vi "Loop_SM.vi"() -> ()   [LabVIEW 2017]
uses:
  ENUM_SM_State.ctl
  ENUM_SM_Action.ctl
  TypeDef/CLUSTER_CMD_WC_Drive.ctl
  TypeDef/ENUM_WC_Drive_DriveMode.ctl
  TypeDef/CLUSTER_Drive_ACT Loop_VBus Data.ctl
  TypeDef/CLUSTER_X and Y.ctl
  TypeDef/CLUSTER_Drive_ACT Loop_Profile Data.ctl
  TypeDef/CLUSTER_Left and Right.ctl
  TypeDef/ENUM_Drive_ACT Loop_Mode.ctl
  TypeDef/CLUSTER_Drive_HW_SRX_Status.ctl
  TypeDef/CLUSTER_4296_SRX_Status.ctl
  TypeDef/CLUSTER_SRX_Status Data.ctl
  TypeDef/CLUSTER_SRX_Encoder Data.ctl
  TypeDef/CLUSTER_SRX_PWM Data.ctl
  TypeDef/CLUSTER_SRX_Analog Data.ctl
  TypeDef/CLUSTER_SRX_Limit Switch Data.ctl
  TypeDef/CLUSTER_SRX_Profile Data.ctl
  <vilib>/Rock Robotics/WPI/ThirdParty/Sensors/navX/_TypeDefs/FRIC_navX_DeviceNumbersTypeDef.ctl
  _SHARE ALL/Global Share All/Global_STOP.vi
  Globals/Global_CMD_Drive.vi
  Global_ACT Write_Data Out.vi
  <vilib>/addons/control/pid/pid.llb/PID (DBL).vi
  Global_SM Write_Data Out.vi
  <vilib>/addons/control/pid/NI_PID_pid.lvlib
panel:
  in  "PID gains Cube Follow":T1={"proportional gain (Kc)"=0.01, "integral time (Ti, min)"=0.0, "derivative time (Td, min)"=0.0} {"derivative time (Td, min)" format="%.3f"; "integral time (Ti, min)" format="%.3f"; "proportional gain (Kc)" format="%.8f"}
  in  "Pixel allowence":dbl=10.0 format="%#_13g"
  in  "Degree allowence":dbl=2.0 format="%#_13g"
  in  "PID gains Lock Angle":T1={"proportional gain (Kc)"=0.01, "integral time (Ti, min)"=0.0, "derivative time (Td, min)"=0.0} {"derivative time (Td, min)" format="%.3f"; "integral time (Ti, min)" format="%.3f"; "proportional gain (Kc)" format="%.8f"}
  in  "MAX sensativity":dbl=1.0
  in  "Max RPM":dbl=10000.0
  in  "MIN sensativity":dbl=0.2
  out "Cycle Time (S)":dbl format="%.3g"
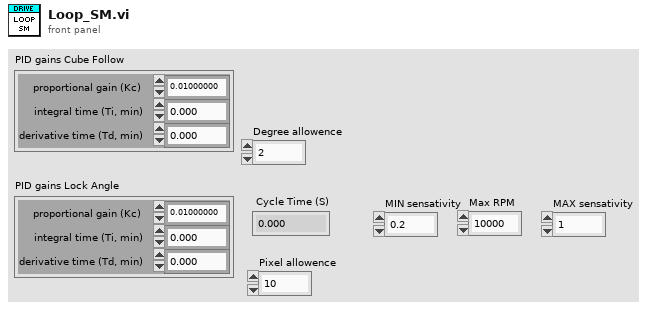
[diagram p1: front panel]
types:
  T1 = cluster{"proportional gain (Kc)":dbl, "integral time (Ti, min)":dbl, "derivative time (Td, min)":dbl}
  T2 = cluster{"Rollover":dbl, "Yaw":dbl, "Cont Yaw":dbl}
  T3 = typedef "CLUSTER_Drive_HW_SRX_Status.ctl" = cluster{"Rear Left":T4, "Rear Right":T4, "Front Left":T4, "Front Right":T4}
  T4 = typedef "CLUSTER_4296_SRX_Status.ctl" = cluster{"Status":T5, "Encoder":T6, "PWM ":T7, "Analog":T8, "Limit Switches":T9, "Profile":T10}
  T5 = typedef "CLUSTER_SRX_Status Data.ctl" = cluster{"Module Enabled":bool, "Current Profile Slot Select":dbl, "Brake is Enabled":bool, "Applied Throttle":dbl, "Current":dbl, "Battery Voltage":dbl, "Sticky Fault - Under Voltage":bool, "Temperature (C)":dbl, "Sticky Fault - Over Temp":bool, "CAN Error":errorcluster, "Control 5 Is Supported":bool}
  T6 = typedef "CLUSTER_SRX_Encoder Data.ctl" = cluster{"Closed Loop Error":dbl, "Sensor Position":dbl, "Sensor Velocity":dbl, "Encoder Position":dbl, "Encoder Velocity":dbl, "Encoder Index Count":dbl, "Encoder A Pin State":bool, "Encoder B Pin State":bool, "Encoder Index Pin State":bool, "Pos Div 8":bool, "Vel Div 4":bool}
  T7 = typedef "CLUSTER_SRX_PWM Data.ctl" = cluster{"Closed Loop Error":dbl, "Pulse Width Position":i32, "Pulse Width Velocity":i32, "Pulse Width Rise To Rise (us)":i32, "Pulse Width Rise To Fall (us)":i32}
  T8 = typedef "CLUSTER_SRX_Analog Data.ctl" = cluster{"Closed Loop Error":dbl, "Analog In":dbl, "Analog In Velocity":dbl}
  T9 = typedef "CLUSTER_SRX_Limit Switch Data.ctl" = cluster{"Forward Limit Switch Closed":bool, "Reverse Limit Switch Closed":bool, "Sticky Fault - Forward Limit":bool, "Sticky Fault - Reverse Limit":bool, "Sticky Fault - Forward Soft Limit":bool, "Sticky Fault - Reverse Soft Limit":bool}
  T10 = typedef "CLUSTER_SRX_Profile Data.ctl" = cluster{"Mot Prof Active Is Under Run":bool, "Mot Prof Active Has Under Run":bool, "Mot Prof Active Is Last":bool, "Mot Prof Active Velocity Only":bool, "Mot Prof Active Is Valid":bool, "Mot Prof Buffer Is Full":bool, "Mot Prof Active Profile Slot Select":i32, "Mot Prof NextID":i32, "Mot Prof Count":i32, "Mot Prof Active Velocity":dbl, "Mot Prof Active Position":dbl, "Mot Prof Output Enable":i32}
  T11 = typedef "ENUM_Drive_ACT Loop_Mode.ctl" = enum16{"Stop", "Position", "VBus", "Profile"}
  T12 = typedef "CLUSTER_Left and Right.ctl" = cluster{"Left":dbl, "Right":dbl}
  T13 = typedef "CLUSTER_CMD_WC_Drive.ctl" = cluster{"Drive_Mode":T14, "VBus":T15, "Profile":T17, "Zero Drive Encoders":bool, "Set Target Position(IN)":dbl, "Target Angle(Degree)":dbl, "Lock Angle":bool, "Zero YAW":bool, "Follow Cubes":bool}
  T14 = typedef "ENUM_WC_Drive_DriveMode.ctl" = enum16{"Motion Profile", "CrossLineAuto", "VBus", "Stop"}
  T15 = typedef "CLUSTER_Drive_ACT Loop_VBus Data.ctl" = cluster{"Drive":T16, "Turbo":bool}
  T16 = typedef "CLUSTER_X and Y.ctl" = cluster{"Steer":dbl, "Throtle":dbl}
  T17 = typedef "CLUSTER_Drive_ACT Loop_Profile Data.ctl" = cluster{"Start":bool}
  T18 = typedef "ENUM_SM_Action.ctl" = enum16{"No Action", "Reset Time", "Reset All", "Drive", "Zero YAW", "Shift", "Calculate Sensitivity"}
  T19 = typedef "ENUM_SM_State.ctl" = enum16{"Startup", "VBus", "VBus Lock Angle", "Idle", "Follow Cube", "Shutdown"}
  T20 = cluster{"Action":T18, "State":T19, "Previous State":T19, "Current Time":timestamp, "Previous Time":timestamp, "Start Time":timestamp, "Target Time (ms)":u32, "Cycle Time(S)":dbl, "CMD_Drive":T13, "VBus Output":T12, "Mode Output":T11, "MQuickStopAccumulator":dbl, "SRX_Status":T3, "Sensitivity":dbl, "NavX Yaw":cluster{"Rollover":dbl, "Yaw":dbl, "Cont Yaw":dbl}, "LockAngle":bool, "Zero YAW":bool, "Target Cube Position (Pixels)":dbl, "Follow Cube":bool}
  T21 = typedef "FRIC_navX_DeviceNumbersTypeDef.ctl" = enum16{"Dev0", "Dev1", "Dev2", "Dev3"}
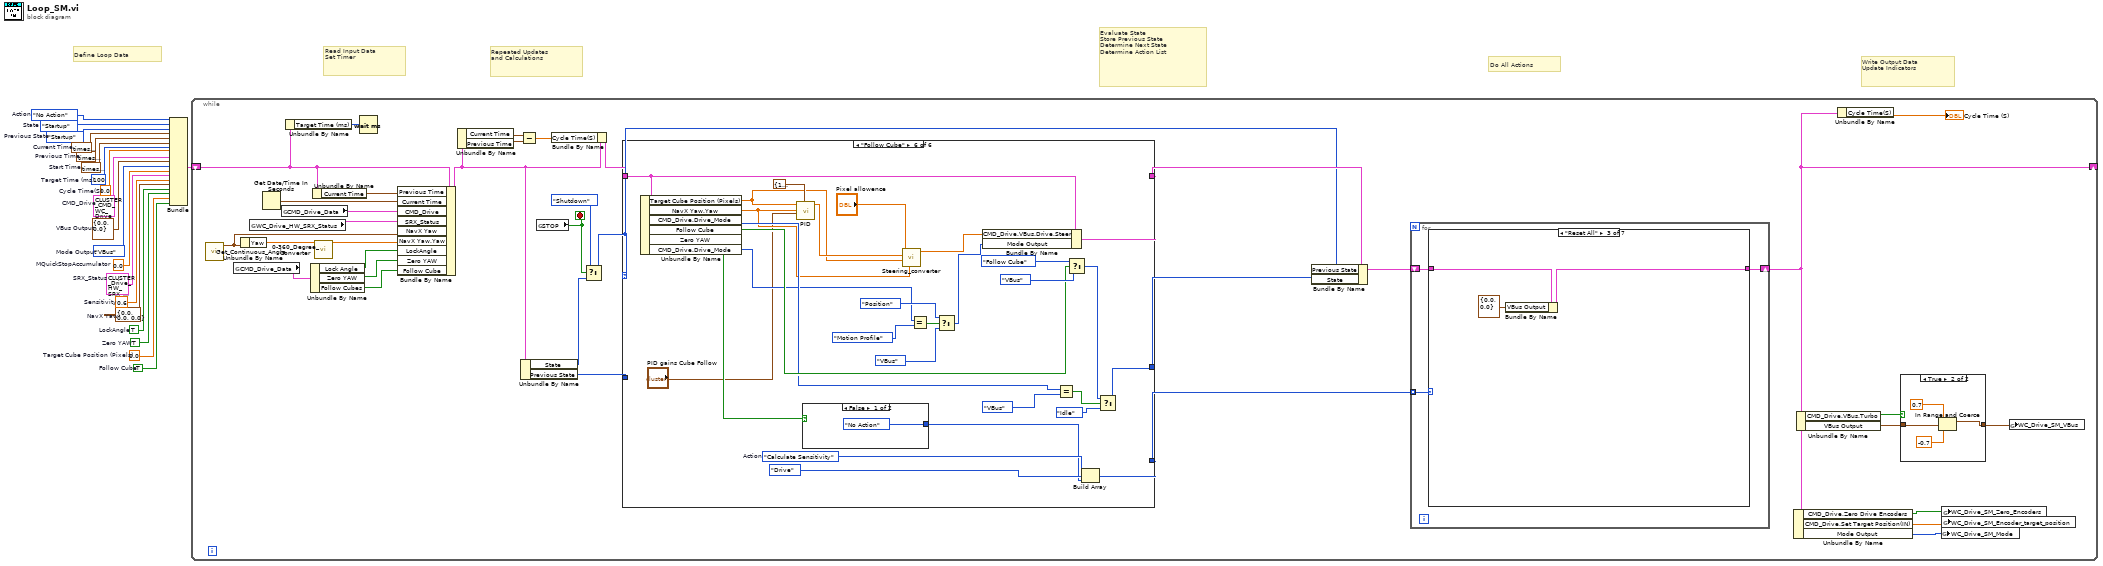
[diagram p0: block diagram]
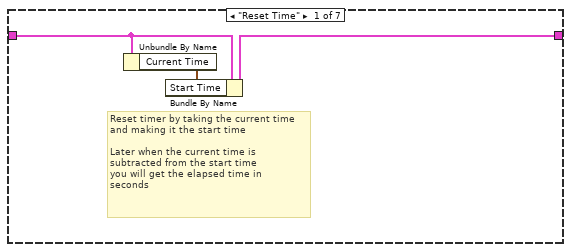
[diagram p3: hidden frame]
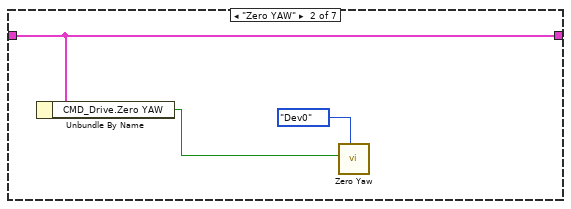
[diagram p4: hidden frame]
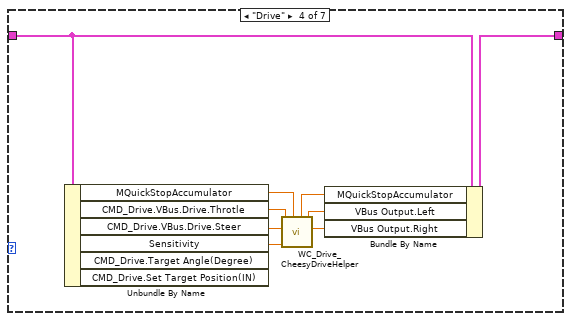
[diagram p5: hidden frame]
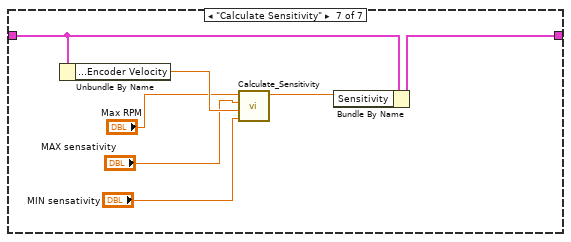
[diagram p8: hidden frame]
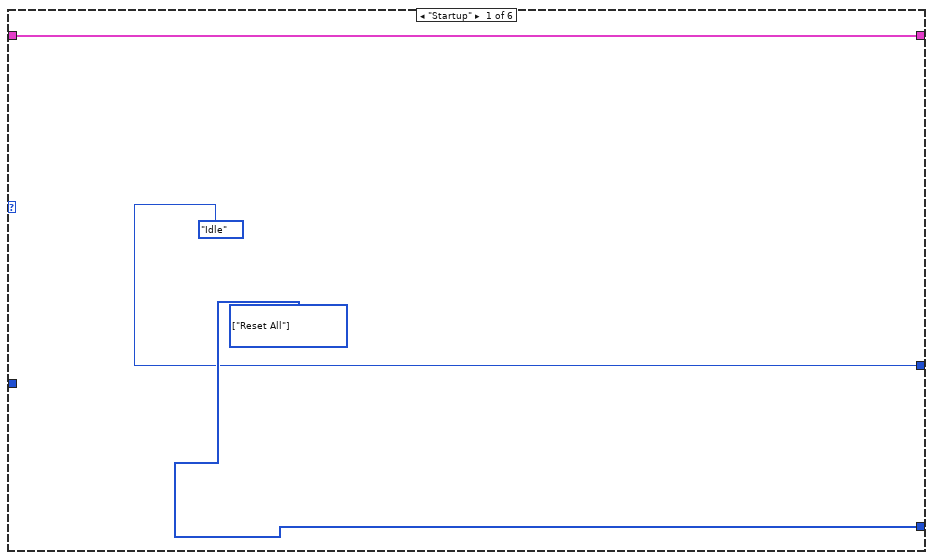
[diagram p9: hidden frame]
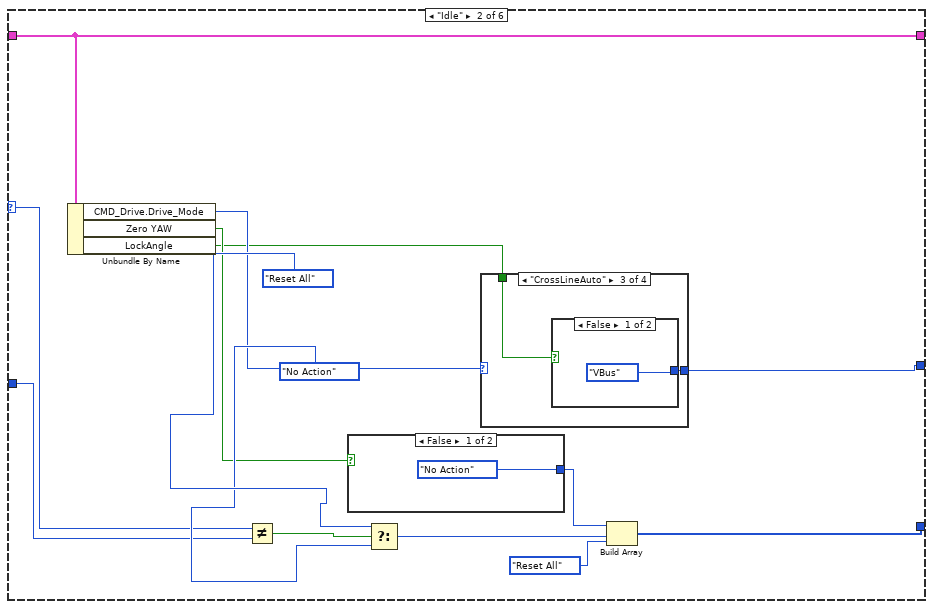
[diagram p10: hidden frame]
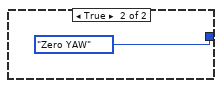
[diagram p11: hidden frame]
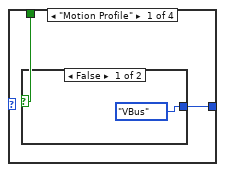
[diagram p12: hidden frame]
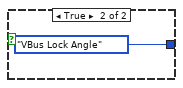
[diagram p13: hidden frame]
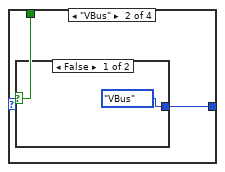
[diagram p14: hidden frame]
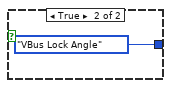
[diagram p15: hidden frame]
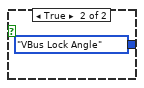
[diagram p16: hidden frame]
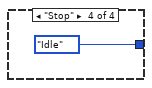
[diagram p17: hidden frame]
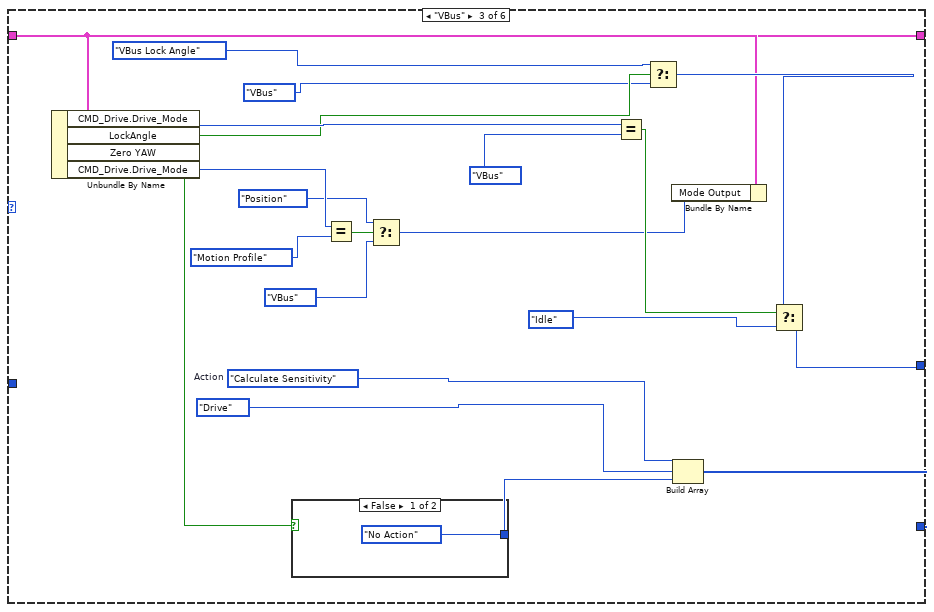
[diagram p18: hidden frame]
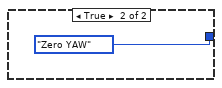
[diagram p19: hidden frame]
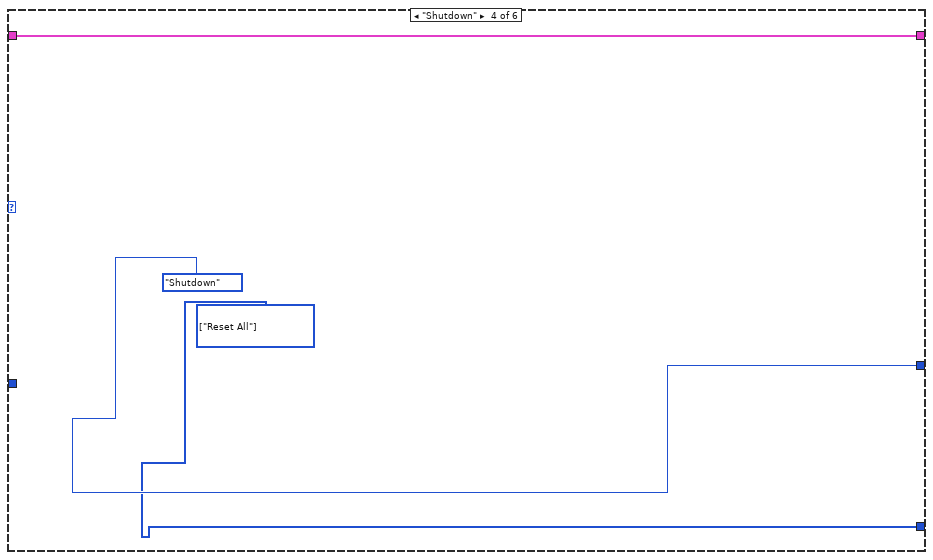
[diagram p20: hidden frame]
diagram:
  w1 = TRUE  # Follow Cube
  w2 = 0.0  # Target Cube Position (Pixels)
  w3 = TRUE  # Zero YAW
  w4 = TRUE  # LockAngle
  w5 = T2 {"Rollover"=0.0, "Yaw"=0.0, "Cont Yaw"=0.0}  # NavX Yaw
  w6 = 0.6  # Sensitivity
  w7 = T3 {"Rear Left"={"Status"={"Module Enabled"=FALSE, "Current Profile Slot Select"=0.0, "Brake is Enabled"=TRUE, "Applied Throttle"=0.0, "Current"=0.0, "Battery Voltage"=12.450000000000001, "Sticky Fault - Under Voltage"=TRUE, "Temperature (C)"=30.645161290322577, "Sticky Fault - Over Temp"=FALSE, "CAN Error"={"status"=FALSE, "code"=0, "source"=""}, "Control 5 Is Supported"=TRUE}, "Encoder"={"Closed Loop Error"=0.0, "Sensor Position"=-847.859619140625, "Sensor Velocity"=0.0, "Encoder Position"=-3472833.0, "Encoder Velocity"=0.0, "Encoder Index Count"=-9452.0, "Encoder A Pin State"=FALSE, "Encoder B Pin State"=FALSE, "Encoder Index Pin State"=FALSE, "Pos Div 8"=FALSE, "Vel Div 4"=FALSE}, "PWM "={"Closed Loop Error"=0.0, "Pulse Width Position"=-3472224, "Pulse Width Velocity"=0, "Pulse Width Rise To Rise (us)"=4187, "Pulse Width Rise To Fall (us)"=1210}, "Analog"={"Closed Loop Error"=0.0, "Analog In"=105.0, "Analog In Velocity"=0.0}, "Limit Switches"={"Forward Limit Switch Closed"=FALSE, "Reverse Limit Switch Closed"=FALSE, "Sticky Fault - Forward Limit"=FALSE, "Sticky Fault - Reverse Limit"=TRUE, "Sticky Fault - Forward Soft Limit"=FALSE, "Sticky Fault - Reverse Soft Limit"=FALSE}, "Profile"={"Mot Prof Active Is Under Run"=FALSE, "Mot Prof Active Has Under Run"=FALSE, "Mot Prof Active Is Last"=FALSE, "Mot Prof Active Velocity Only"=FALSE, "Mot Prof Active Is Valid"=FALSE, "Mot Prof Buffer Is Full"=FALSE, "Mot Prof Active Profile Slot Select"=0, "Mot Prof NextID"=0, "Mot Prof Count"=0, "Mot Prof Active Velocity"=0.0, "Mot Prof Active Position"=0.0, "Mot Prof Output Enable"=0}}, "Rear Right"={"Status"={"Module Enabled"=FALSE, "Current Profile Slot Select"=0.0, "Brake is Enabled"=TRUE, "Applied Throttle"=0.0, "Current"=0.125, "Battery Voltage"=12.4, "Sticky Fault - Under Voltage"=TRUE, "Temperature (C)"=27.41935483870968, "Sticky Fault - Over Temp"=FALSE, "CAN Error"={"status"=FALSE, "code"=0, "source"=""}, "Control 5 Is Supported"=TRUE}, "Encoder"={"Closed Loop Error"=0.0, "Sensor Position"=-228.95263671875, "Sensor Velocity"=0.0, "Encoder Position"=937790.0, "Encoder Velocity"=0.0, "Encoder Index Count"=2928.0, "Encoder A Pin State"=FALSE, "Encoder B Pin State"=TRUE, "Encoder Index Pin State"=TRUE, "Pos Div 8"=FALSE, "Vel Div 4"=FALSE}, "PWM "={"Closed Loop Error"=0.0, "Pulse Width Position"=937817, "Pulse Width Velocity"=0, "Pulse Width Rise To Rise (us)"=4128, "Pulse Width Rise To Fall (us)"=3960}, "Analog"={"Closed Loop Error"=0.0, "Analog In"=103.0, "Analog In Velocity"=0.0}, "Limit Switches"={"Forward Limit Switch Closed"=FALSE, "Reverse Limit Switch Closed"=FALSE, "Sticky Fault - Forward Limit"=FALSE, "Sticky Fault - Reverse Limit"=FALSE, "Sticky Fault - Forward Soft Limit"=FALSE, "Sticky Fault - Reverse Soft Limit"=FALSE}, "Profile"={"Mot Prof Active Is Under Run"=FALSE, "Mot Prof Active Has Under Run"=FALSE, "Mot Prof Active Is Last"=FALSE, "Mot Prof Active Velocity Only"=FALSE, "Mot Prof Active Is Valid"=FALSE, "Mot Prof Buffer Is Full"=FALSE, "Mot Prof Active Profile Slot Select"=0, "Mot Prof NextID"=0, "Mot Prof Count"=0, "Mot Prof Active Velocity"=0.0, "Mot Prof Active Position"=0.0, "Mot Prof Output Enable"=0}}, "Front Left"={"Status"={"Module Enabled"=FALSE, "Current Profile Slot Select"=0.0, "Brake is Enabled"=TRUE, "Applied Throttle"=0.0, "Current"=0.0, "Battery Voltage"=12.4, "Sticky Fault - Under Voltage"=TRUE, "Temperature (C)"=28.709677419354833, "Sticky Fault - Over Temp"=FALSE, "CAN Error"={"status"=FALSE, "code"=0, "source"=""}, "Control 5 Is Supported"=TRUE}, "Encoder"={"Closed Loop Error"=0.0, "Sensor Position"=0.0, "Sensor Velocity"=0.0, "Encoder Position"=0.0, "Encoder Velocity"=0.0, "Encoder Index Count"=0.0, "Encoder A Pin State"=TRUE, "Encoder B Pin State"=TRUE, "Encoder Index Pin State"=TRUE, "Pos Div 8"=FALSE, "Vel Div 4"=FALSE}, "PWM "={"Closed Loop Error"=0.0, "Pulse Width Position"=0, "Pulse Width Velocity"=0, "Pulse Width Rise To Rise (us)"=0, "Pulse Width Rise To Fall (us)"=0}, "Analog"={"Closed Loop Error"=0.0, "Analog In"=105.0, "Analog In Velocity"=0.0}, "Limit Switches"={"Forward Limit Switch Closed"=FALSE, "Reverse Limit Switch Closed"=FALSE, "Sticky Fault - Forward Limit"=FALSE, "Sticky Fault - Reverse Limit"=FALSE, "Sticky Fault - Forward Soft Limit"=FALSE, "Sticky Fault - Reverse Soft Limit"=FALSE}, "Profile"={"Mot Prof Active Is Under Run"=FALSE, "Mot Prof Active Has Under Run"=FALSE, "Mot Prof Active Is Last"=FALSE, "Mot Prof Active Velocity Only"=FALSE, "Mot Prof Active Is Valid"=FALSE, "Mot Prof Buffer Is Full"=FALSE, "Mot Prof Active Profile Slot Select"=0, "Mot Prof NextID"=0, "Mot Prof Count"=0, "Mot Prof Active Velocity"=0.0, "Mot Prof Active Position"=0.0, "Mot Prof Output Enable"=0}}, "Front Right"={"Status"={"Module Enabled"=FALSE, "Current Profile Slot Select"=0.0, "Brake is Enabled"=TRUE, "Applied Throttle"=0.0, "Current"=0.0, "Battery Voltage"=12.35, "Sticky Fault - Under Voltage"=TRUE, "Temperature (C)"=26.77419354838709, "Sticky Fault - Over Temp"=FALSE, "CAN Error"={"status"=FALSE, "code"=0, "source"=""}, "Control 5 Is Supported"=TRUE}, "Encoder"={"Closed Loop Error"=0.0, "Sensor Position"=0.0, "Sensor Velocity"=0.0, "Encoder Position"=0.0, "Encoder Velocity"=0.0, "Encoder Index Count"=0.0, "Encoder A Pin State"=TRUE, "Encoder B Pin State"=TRUE, "Encoder Index Pin State"=TRUE, "Pos Div 8"=FALSE, "Vel Div 4"=FALSE}, "PWM "={"Closed Loop Error"=0.0, "Pulse Width Position"=0, "Pulse Width Velocity"=0, "Pulse Width Rise To Rise (us)"=0, "Pulse Width Rise To Fall (us)"=0}, "Analog"={"Closed Loop Error"=0.0, "Analog In"=102.0, "Analog In Velocity"=0.0}, "Limit Switches"={"Forward Limit Switch Closed"=FALSE, "Reverse Limit Switch Closed"=FALSE, "Sticky Fault - Forward Limit"=FALSE, "Sticky Fault - Reverse Limit"=TRUE, "Sticky Fault - Forward Soft Limit"=FALSE, "Sticky Fault - Reverse Soft Limit"=FALSE}, "Profile"={"Mot Prof Active Is Under Run"=FALSE, "Mot Prof Active Has Under Run"=FALSE, "Mot Prof Active Is Last"=FALSE, "Mot Prof Active Velocity Only"=FALSE, "Mot Prof Active Is Valid"=FALSE, "Mot Prof Buffer Is Full"=FALSE, "Mot Prof Active Profile Slot Select"=0, "Mot Prof NextID"=0, "Mot Prof Count"=0, "Mot Prof Active Velocity"=0.0, "Mot Prof Active Position"=0.0, "Mot Prof Output Enable"=0}}}  # SRX_Status
  w8 = 0.0  # MQuickStopAccumulator
  w9 = ENUM_Drive_ACT_Loop_Mode."VBus"  # Mode Output
  w10 = T12 {"Left"=0.0, "Right"=0.0}  # VBus Output
  w11 = T13 {"Drive_Mode"=enum."Motion Profile", "VBus"={"Drive"={"Steer"=0.0, "Throtle"=0.0}, "Turbo"=FALSE}, "Profile"={"Start"=FALSE}, "Zero Drive Encoders"=FALSE, "Set Target Position(IN)"=0.0, "Target Angle(Degree)"=0.0, "Lock Angle"=FALSE, "Zero YAW"=FALSE, "Follow Cubes"=FALSE}  # CMD_Drive
  w12 = ENUM_SM_Action."No Action"  # Action
  w13 = 0.0  # Cycle Time(S)
  w14 = ENUM_SM_State."Startup"  # Previous State
  w15 = timestamp(0 s since 1904-01-01)  # Previous Time
  w16 = u32 100  # Target Time (ms)
  w17 = timestamp(0 s since 1904-01-01)  # Start Time
  w18 = timestamp(0 s since 1904-01-01)  # Current Time
  w19 = ENUM_SM_State."Startup"  # State
  # "Define Loop Data"
  # "Repeated Updates\nand Calculations"
  # "Read Input Data\nSet Timer"
  # "Evaluate State\nStore Previous State\nDetermine Next State\nDetermine Action List"
  # "Do All Actions"
  # "Write Output Data\nUpdate Indicators"
  n1 = Bundle("Action"=w12, "State"=w19, "Previous State"=w14, "Current Time"=w18, "Previous Time"=w15, "Start Time"=w17, "Target Time (ms)"=w16, "Cycle Time(S)"=w13, "CMD_Drive"=w11, "VBus Output"=w10, "Mode Output"=w9, "MQuickStopAccumulator"=w8, "SRX_Status"=w7, "Sensitivity"=w6, "NavX Yaw"=w5, "LockAngle"=w4, "Zero YAW"=w3, "Target Cube Position (Pixels)"=w2, "Follow Cube"=w1) -> (w20:T20)  [unwired: 1 in]
  n2 = while {
    shift-right: [w35] -> _
    shift-left: w20 -> [w46]
    stop <- w51 stop-if-true
    n3 = call <vilib>:"Get_Continuous_Angle.vi"() -> ("Continuous Angle"=w31:T2)  [unwired: 11 in]
    n4 = global read "Global_CMD_Drive.vi" "CMD_Drive_Data"() -> (w26:T13)
    n5 = Unbundle By Name(w31) -> ("Yaw"=w30:dbl)
    n6 = global read "Global_ACT Write_Data Out.vi" "WC_Drive_HW_SRX_Status"() -> (w32:T3)
    n7 = Get Date/Time In Seconds() -> (seconds since 1Jan1904=w55:timestamp)
    n8 = global read "Global_CMD_Drive.vi" "CMD_Drive_Data"() -> (w36:T13)
    n9 = Unbundle By Name(w46) -> ("Target Time (ms)"=w48:u32)
    n10 = Unbundle By Name(w26) -> ("Lock Angle"=w25:bool, "Zero YAW"=w24:bool, "Follow Cubes"=w21:bool)
    n11 = Unbundle By Name(w46) -> ("Current Time"=w47:timestamp)
    n12 = call "0-360_Degree_Converter.vi"("Yaw in"=w30) -> ("Yaw out"=w27:dbl)  [unwired: 10 in]
    n13 = Wait (ms)(milliseconds to wait=w48) -> ()  [unwired: 1 out]
    n14 = Bundle By Name(cluster=w46, "Previous Time"=w47, "Current Time"=w55, "CMD_Drive"=w36, "SRX_Status"=w32, "NavX Yaw"=w31, "NavX Yaw.Yaw"=w27, "LockAngle"=w25, "Zero YAW"=w24, "Follow Cube"=w21) -> (w28:T20)
    n15 = Unbundle By Name(w28) -> ("Current Time"=w41:timestamp, "Previous Time"=w42:timestamp)
    n16 = Subtract(x=w41, y=w42) -> (x-y=w39:dbl)
    n17 = Unbundle By Name(w28) -> ("State"=w49:T19, "Previous State"=w45:T19)
    n18 = global read "Global_STOP.vi" "STOP"() -> (w51:bool)
    n19 = Bundle By Name(cluster=w28, "Cycle Time(S)"=w39) -> (w40:T20)
    n20 = Select(t=ENUM_SM_State."Shutdown" ("State"), s=w51, f=w49) -> (s? t:f=w44:T19)
    n21 = case shown="\"Follow Cube\"" w44 {
      selector: w44 -> [_ w101 _ _ _ _]
      tunnel: w40 -> [w93 w107 w125 w149 w174 w205]
      tunnel: [w93 w107 w124 w149 w178 w209] -> w53
      tunnel: [ENUM_SM_State."Idle" ("State") w98 w144 ENUM_SM_State."Shutdown" ("State") w166 w198] -> w52
      tunnel: [w92 w102 w140 w147 w175 w206] -> w38
      tunnel: w45 -> [_ w100 _ _ _ _]
      frame "Startup" {
        w92 = T18[] [enum."Reset All"] items=["No Action", "Reset Time", "Reset All", "Drive", "Zero YAW", "Shift", "Calculate Sensitivity"] ("Actions")
      }
      frame "Idle" {
        n22 = Unbundle By Name(w107) -> ("CMD_Drive.Drive_Mode"=w99:T14, "Zero YAW"=w96:bool, "LockAngle"=w95:bool)
        n23 = Not Equal?(x=w101, y=w100) -> (x != y?=w106:bool)
        n24 = case shown="False" w96 {
          tunnel: [ENUM_SM_Action."No Action" ("element") ENUM_SM_Action."Zero YAW" ("element")] -> w97
          frame False {
          }
          frame True {
          }
        }
        n25 = Select(t=ENUM_SM_Action."Reset All" ("Action"), s=w106, f=ENUM_SM_Action."No Action" ("Action")) -> (s? t:f=w105:T18)
        n26 = case shown="\"CrossLineAuto\"" w99 {
          tunnel: [w111 w115 w119 ENUM_SM_State."Idle" ("State")] -> w98
          tunnel: w95 -> [w110 w114 w118 _]
          frame "Motion Profile" {
            n27 = case shown="False" w110 {
              tunnel: [ENUM_SM_State."VBus" ("State") ENUM_SM_State."VBus Lock Angle" ("State")] -> w111
              frame False {
              }
              frame True {
              }
            }
          }
          frame "VBus" {
            n28 = case shown="False" w114 {
              tunnel: [ENUM_SM_State."VBus" ("State") ENUM_SM_State."VBus Lock Angle" ("State")] -> w115
              frame False {
              }
              frame True {
              }
            }
          }
          frame "CrossLineAuto" {
            n29 = case shown="False" w118 {
              tunnel: [ENUM_SM_State."VBus" ("State") ENUM_SM_State."VBus Lock Angle" ("State")] -> w119
              frame False {
              }
              frame True {
              }
            }
          }
          frame "Stop" {
          }
        }
        n30 = Build Array(w97, w105, ENUM_SM_Action."Reset All" ("element")) -> (w102:T18[])
      }
      frame "VBus" {
        w141 = ENUM_SM_Action."Calculate Sensitivity"  # Action
        n31 = Unbundle By Name(w125) -> ("CMD_Drive.Drive_Mode"=w143:T14, "LockAngle"=w135:bool, "Zero YAW"=w132:bool, "CMD_Drive.Drive_Mode"=w128:T14)
        n32 = case shown="False" w132 {
          tunnel: [ENUM_SM_Action."No Action" ("element") ENUM_SM_Action."Zero YAW" ("element")] -> w131
          frame False {
          }
          frame True {
          }
        }
        n33 = Equal?(x=w128, y=ENUM_WC_Drive_DriveMode."Motion Profile" ("CMD_Drive.Drive_Mode")) -> (x = y?=w130:bool)
        n34 = Select(t=ENUM_Drive_ACT_Loop_Mode."Position" ("WC_Drive_SM_Mode"), s=w130, f=ENUM_Drive_ACT_Loop_Mode."VBus" ("WC_Drive_SM_Mode")) -> (s? t:f=w123:T11)
        n35 = Equal?(x=w143, y=ENUM_WC_Drive_DriveMode."VBus" ("CMD_Drive_Mode")) -> (x = y?=w142:bool)
        n36 = Select(t=ENUM_SM_State."VBus Lock Angle" ("State"), s=w135, f=ENUM_SM_State."VBus" ("State")) -> (s? t:f=w136:T19)
        n37 = Bundle By Name(cluster=w125, "Mode Output"=w123) -> (w124:T20)
        n38 = Build Array(w141, ENUM_SM_Action."Drive" ("element"), w131) -> (w140:T18[])
        n39 = Select(t=w136, s=w142, f=ENUM_SM_State."Idle" ("State")) -> (s? t:f=w144:T19)
      }
      frame "Shutdown" {
        w147 = T18[] [enum."Reset All"] items=["No Action", "Reset Time", "Reset All", "Drive", "Zero YAW", "Shift", "Calculate Sensitivity"] ("Actions")
      }
      frame "VBus Lock Angle" {
        w177 = ENUM_SM_Action."Calculate Sensitivity"  # Action
        n40 = Unbundle By Name(w174) -> ("CMD_Drive.Target Angle(Degree)"=w157:dbl, "NavX Yaw.Yaw"=w160:dbl, "CMD_Drive.Drive_Mode"=w164:T14, "LockAngle"=w165:bool, "Zero YAW"=w158:bool, "CMD_Drive.Drive_Mode"=w152:T14)
        n41 = call-poly <vilib>:"PID.vi"("output range"=cluster{"output high":dbl, "output low":dbl} {"output high"=1.0, "output low"=-1.0}, "PID gains"="PID gains Lock Angle", "process variable"=w160, "setpoint"=w157) -> ("output"=w161:dbl)  [unwired: 6 in, 1 out]
        n42 = case shown="False" w158 {
          tunnel: [ENUM_SM_Action."No Action" ("element") ENUM_SM_Action."Zero YAW" ("element")] -> w159
          frame False {
          }
          frame True {
          }
        }
        n43 = call "Steering_converter.vi"("Yaw"=w160, "setpoint"=w157, "output"=w161, "Degree allowence"="Degree allowence") -> ("Steer"=w162:dbl)  [unwired: 7 in]
        n44 = Equal?(x=w152, y=ENUM_WC_Drive_DriveMode."Motion Profile" ("CMD_Drive.Drive_Mode")) -> (x = y?=w156:bool)
        n45 = Select(t=ENUM_Drive_ACT_Loop_Mode."Position" ("WC_Drive_SM_Mode"), s=w156, f=ENUM_Drive_ACT_Loop_Mode."VBus" ("WC_Drive_SM_Mode")) -> (s? t:f=w151:T11)
        n46 = Bundle By Name(cluster=w174, "CMD_Drive.VBus.Drive.Steer"=w162, "Mode Output"=w151) -> (w178:T20)
        n47 = Equal?(x=w164, y=ENUM_WC_Drive_DriveMode."VBus" ("CMD_Drive_Mode")) -> (x = y?=w172:bool)
        n48 = Select(t=ENUM_SM_State."VBus Lock Angle" ("State"), s=w165, f=ENUM_SM_State."VBus" ("State")) -> (s? t:f=w169:T19)
        n49 = Build Array(w177, ENUM_SM_Action."Drive" ("element"), w159) -> (w175:T18[])
        n50 = Select(t=w169, s=w172, f=ENUM_SM_State."Idle" ("State")) -> (s? t:f=w166:T19)
      }
      frame "Follow Cube" {
        w208 = ENUM_SM_Action."Calculate Sensitivity"  # Action
        n51 = Unbundle By Name(w205) -> ("Target Cube Position (Pixels)"=w189:dbl, "NavX Yaw.Yaw"=w192:dbl, "CMD_Drive.Drive_Mode"=w196:T14, "Follow Cube"=w197:bool, "Zero YAW"=w190:bool, "CMD_Drive.Drive_Mode"=w184:T14)
        n52 = call-poly <vilib>:"PID.vi"("output range"=cluster{"output high":dbl, "output low":dbl} {"output high"=1.0, "output low"=-1.0}, "PID gains"="PID gains Cube Follow", "process variable"=w192, "setpoint"=w189) -> ("output"=w193:dbl)  [unwired: 6 in, 1 out]
        n53 = case shown="False" w190 {
          tunnel: [ENUM_SM_Action."No Action" ("element") ENUM_SM_Action."Zero YAW" ("element")] -> w191
          frame False {
          }
          frame True {
          }
        }
        n54 = call "Steering_converter.vi"("Yaw"=w192, "setpoint"=w189, "output"=w193, "Degree allowence"="Pixel allowence") -> ("Steer"=w194:dbl)  [unwired: 7 in]
        n55 = Equal?(x=w184, y=ENUM_WC_Drive_DriveMode."Motion Profile" ("CMD_Drive.Drive_Mode")) -> (x = y?=w188:bool)
        n56 = Select(t=ENUM_Drive_ACT_Loop_Mode."Position" ("WC_Drive_SM_Mode"), s=w188, f=ENUM_Drive_ACT_Loop_Mode."VBus" ("WC_Drive_SM_Mode")) -> (s? t:f=w183:T11)
        n57 = Bundle By Name(cluster=w205, "CMD_Drive.VBus.Drive.Steer"=w194, "Mode Output"=w183) -> (w209:T20)
        n58 = Equal?(x=w196, y=ENUM_WC_Drive_DriveMode."VBus" ("CMD_Drive_Mode")) -> (x = y?=w204:bool)
        n59 = Select(t=ENUM_SM_State."Follow Cube" ("State"), s=w197, f=ENUM_SM_State."VBus" ("State")) -> (s? t:f=w201:T19)
        n60 = Build Array(w208, ENUM_SM_Action."Drive" ("element"), w191) -> (w206:T18[])
        n61 = Select(t=w201, s=w204, f=ENUM_SM_State."Idle" ("State")) -> (s? t:f=w198:T19)
      }
    }
    n62 = Bundle By Name(cluster=w53, "Previous State"=w44, "State"=w52) -> (w54:T20)
    n63 = for {
      tunnel: w38 -> [w63] mode=indexing
      shift-right: [w62] -> w35
      shift-left: w54 -> [w61]
      n64 = case shown="\"Reset All\"" w63 {
        tunnel: w61 -> [w66 w68 w72 w81 w82 w83 w90]
        tunnel: [w65 w68 w71 w80 w82 w83 w89] -> w62
        frame "Reset Time" {
          # "Reset timer by taking the current time\nand making it the start time\n\nLater when the current time is \nsubtracted from the start time\nyou will get the elapsed time in \nseconds"
          n65 = Unbundle By Name(w66) -> ("Current Time"=w64:timestamp)
          n66 = Bundle By Name(cluster=w66, "Start Time"=w64) -> (w65:T20)
        }
        frame "Zero YAW" {
          n67 = Unbundle By Name(w68) -> ("CMD_Drive.Zero YAW"=w67:bool)
          n68 = call <vilib>:"Zero Yaw.vi"("Device Number"=FRIC_navX_DeviceNumbersTypeDef."Dev0", "Zero"=w67) -> ()  [unwired: 10 in]
        }
        frame "Reset All" {
          n69 = Bundle By Name(cluster=w72, "VBus Output"=T12 {"Left"=0.0, "Right"=0.0}) -> (w71:T20)
        }
        frame "Drive" {
          n70 = Unbundle By Name(w81) -> ("MQuickStopAccumulator"=w78:dbl, "CMD_Drive.VBus.Drive.Throtle"=w77:dbl, "CMD_Drive.VBus.Drive.Steer"=w76:dbl, "Sensitivity"=w75:dbl)  [unwired: 2 out]
          n71 = call "WC_Drive_CheesyDriveHelper.vi"("MQuickStopAccumulator"=w78, "KTurnSensitivity"=w75, "Steer"=w76, "Throttle"=w77) -> ("RightPwm Out"=w73:dbl, "LeftPwm Out"=w74:dbl, "MQuickStopAccumulator Out"=w79:dbl)  [unwired: 5 in]
          n72 = Bundle By Name(cluster=w81, "MQuickStopAccumulator"=w79, "VBus Output.Left"=w74, "VBus Output.Right"=w73) -> (w80:T20)
        }
        frame "No Action" {
        }
        frame "Shift" {
        }
        frame "Calculate Sensitivity" {
          n73 = Unbundle By Name(w90) -> ("SRX_Status.Rear Right.Encoder.Encoder Velocity"=w87:dbl)
          n74 = call "Calculate_Sensitivity.vi"("Min Sensitivity"="MIN sensativity", "Current RPM"=w87, "Max Sensitivity"="MAX sensativity", "Max RPM"="Max RPM") -> ("Sensitivity"=w88:dbl)  [unwired: 7 in]
          n75 = Bundle By Name(cluster=w90, "Sensitivity"=w88) -> (w89:T20)
        }
      }
    }
    n76 = Unbundle By Name(w35) -> ("CMD_Drive.Zero Drive Encoders"=w22:bool, "CMD_Drive.Set Target Position(IN)"=w23:dbl, "Mode Output"=w29:T11)
    n77 = Unbundle By Name(w35) -> ("CMD_Drive.VBus.Turbo"=w33:bool, "VBus Output"=w37:T12)
    n78 = Unbundle By Name(w35) -> ("Cycle Time(S)"=→"Cycle Time (S)":dbl)
    n79 = case shown="True" w33 {
      tunnel: w37 -> [w56 w60]
      tunnel: [w56 w57] -> w34
      frame False {
      }
      frame True {
        n80 = In Range and Coerce(upper limit=0.7, x=w60, lower limit=-0.7) -> (coerced(x)=w57:T12)  [unwired: 1 out]
      }
    }
    n81 = global write "Global_SM Write_Data Out.vi" "WC_Drive_SM_Mode"(w29) -> ()
    n82 = global write "Global_SM Write_Data Out.vi" "WC_Drive_SM_Zero_Encoders"(w22) -> ()
    n83 = global write "Global_SM Write_Data Out.vi" "WC_Drive_SM_Encoder_target_position"(w23) -> ()
    n84 = global write "Global_SM Write_Data Out.vi" "WC_Drive_SM_VBus"(w34) -> ()
  }
